vi "Close.vi"(11 "CD in":refnum<class "Template.lvclass">) -> (0 "error out":errorcluster, 3 "CD out":refnum<class "Template.lvclass">)   [LabVIEW 2026, in "Template Plugin.lvlib" / "Template.lvclass"]
uses:
  Template.lvclass
  Template.lvclass/Template.ctl
  <userlib>/NIVS Inline Async API (Express)/_VS Inline Async API (Express)/VS Inline Async API (Express)/VS Inline Async API (Express).lvclass
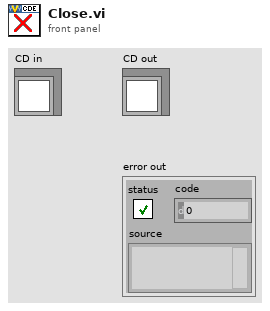
[diagram p1: front panel]
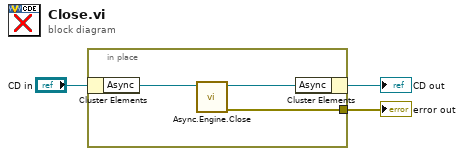
[diagram p0: block diagram]
diagram:
  n1 = in-place {
    in-place-border: [w6] -> w1
    n2 = in-place-cluster #1("CD in") -> ("Async"=w5:refnum<class "VS Inline Async API (Express).lvclass">)
    n3 = call <userlib>:"Async.Engine.Close.vi"("Async in"=w5) -> ("error out"=w6:errorcluster, "Async out"=w4:refnum<class "VS Inline Async API (Express).lvclass">)  [unwired: 9 in]
    n4 = in-place-cluster #1("Async"=w4) -> (→"CD out":refnum<class "Template.lvclass">)
  }
  "error out" <- w1
